vi "BinSearchVIwarmcold.vi"(8 "X0":sgl=0.5, 11 "Ring":i16(ring) items=["Warm", "Cold"]) -> (3 "Xpot":sgl)   [LabVIEW 2019]
uses:
  <vilib>/Platform/TimedLoop/XDataNode/timing_clust.ctl
  <vilib>/Platform/TimedLoop/XDataNode/nitl_modes.ctl
  <vilib>/Platform/TimedLoop/XDataNode/wakeup.ctl
  <vilib>/rvi/Emulation/niFpgaGetClockAttributes.vi
  <vilib>/rvi/Emulation/niFpgaSctlEmulationGetInTimedLoop.vi
  <vilib>/rvi/Emulation/niFpgaEmulationReportErrorSimple.vi
  <vilib>/rvi/Emulation/niFpgaCriticalErrorInLSC.vi
  <vilib>/Platform/TimedLoop/XDataNode/XDataNode.xnode
  <vilib>/Platform/TimedLoop/XDataNode/XDNodeRunTimeDep.lvlib
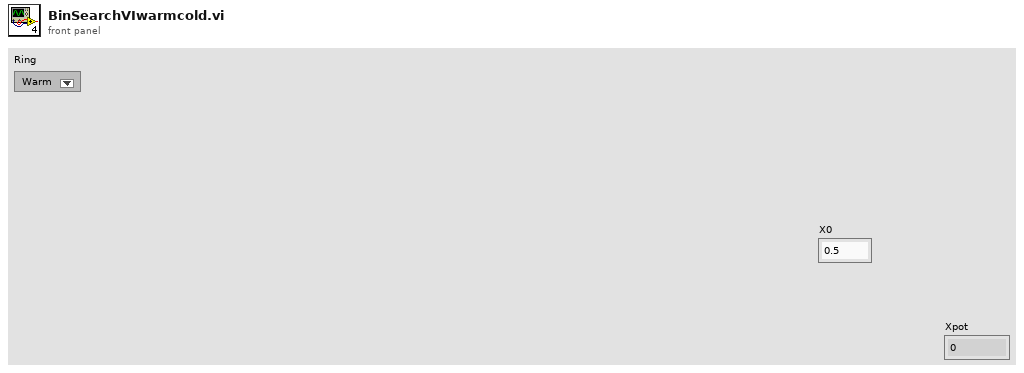
[diagram p1: front panel]
types:
  T1 = typedef "XDNodeRunTimeDep.lvlib/timing_clust.ctl" = cluster{"Expected End [f-1]":u64, "Actual End [f-1]":u64, "Finished Late? [f-1]":bool, "Expected End [i-1]":u64, "Actual End [i-1]":u64, "Finished Late? [i-1]":bool, "Expected Start [i]":u64, "Actual Start [i]":u64, "Expected Start [f]":u64, "Actual Start [f]":u64, "Source Name":string, "Structure Name":string, "Period":i64, "Deadline":i64, "Offset":i64, "Start":i64, "Priority":i32, "Timeout":i32, "Mode":T2, "Wakeup Reason":T3, "Error":errorcluster, "Source Type":string, "Secondary Source Type":string, "Global End Time":u64, "Global Start Time":u64, "Frame Duration":u64, "Iteration Duration":u64, "Assigned CPU":i32, "I/O Scan Engine Mode":u32}
  T2 = typedef "XDNodeRunTimeDep.lvlib/nitl_modes.ctl" = enum32{"No Change", "Process missed periods, maintain original phase", "Discard missed periods, maintain original phase", "Process missed periods, ignore original phase", "Discard missed periods, ignore original phase"}
  T3 = typedef "XDNodeRunTimeDep.lvlib/wakeup.ctl" = enum32{"Normal", "Aborted", "Asynchronous wakeup", "Timing source error", "Timed loop error", "Timeout"}
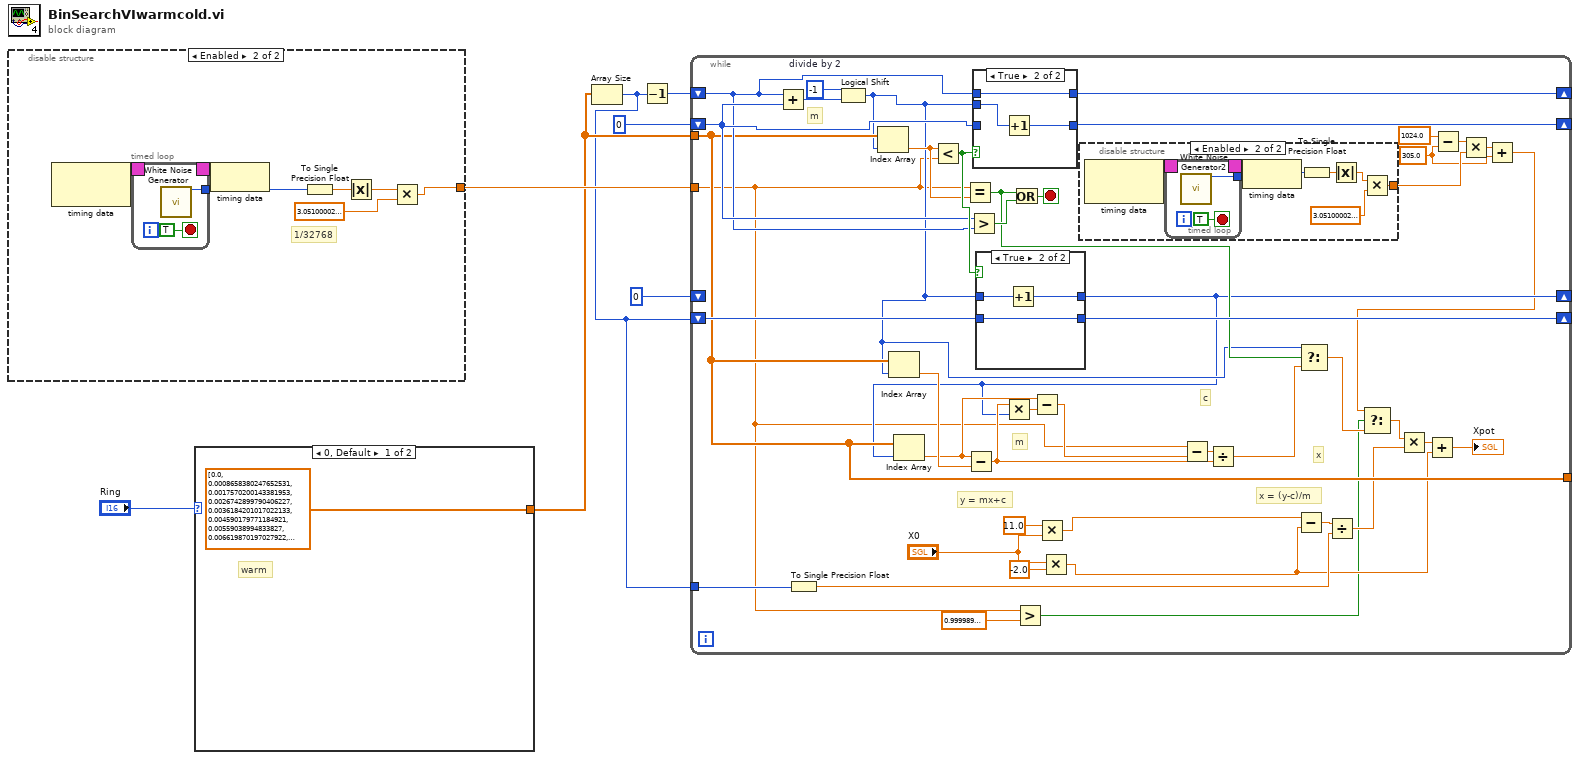
[diagram p0: block diagram]
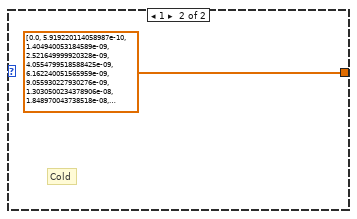
[diagram p2: hidden frame]
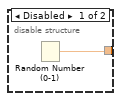
[diagram p3: hidden frame]
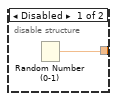
[diagram p4: hidden frame]
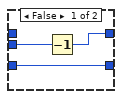
[diagram p6: hidden frame]
diagram:
  n1 = disable-structure shown="Enabled" {
    disable-tunnel: [w8 w11] -> w4
    frame Disabled {
      n2 = Random Number (0-1)() -> (number: 0 to 1=w8:dbl)
    }
    frame Enabled {
      # "1/32768"
      n3 = node-c288() -> (w10:T1)  [unwired: 1 in]
      n4 = timed-loop {
        timing: w10 -> [_]
        timing-out: [_] -> w9
        tunnel: [w17] -> w15
        stop <- TRUE stop-if-true
        n5 = call "White Noise Generator"() -> ("white noise out"=w17:i16)  [unwired: 15 in]
      }
      n6 = node-c288(w9) -> ()
      n7 = To Single Precision Float(number=w15) -> (single precision float=w13:sgl)
      n8 = Absolute Value(x=w13) -> (abs(x)=w12:sgl)
      n9 = Multiply(x=w12, y=sgl 3.051e-05) -> (x*y=w11:sgl)
    }
  }
  n10 = case shown="0, Default" "Ring" {
    tunnel: [sgl[] [0.0, 0.000865838, 0.00175702, 0.00267429, 0.00361842, 0.00459018, 0.00559039, 0.00661987, 0.0076795, 0.00877014, 0.00989271, 0.0110481, 0.0122374, 0.0134615, 0.0147214, 0.0160181, 0.0173529, 0.0187267, 0.0201407, 0.0215961, 0.0230942, 0.0246361, 0.0262231, 0.0278565, 0.0295378, 0.0312683, 0.0330498, 0.0348832, 0.0367683, 0.0387052, 0.0406935, 0.0427329, 0.044823, 0.0469636, 0.0491541, 0.0513939, 0.0536825, 0.0560193, 0.0584036, 0.0608346, 0.0633115, 0.0658336, 0.0683999, 0.0710095, 0.0736616, 0.076355, 0.0790889, 0.0818621, 0.0846736, 0.0875224, 0.0904072, 0.0933269, 0.0962805, 0.0992667, 0.102284, 0.105332, 0.108409, 0.111514, 0.114646, 0.117803, 0.120985, 0.12419, 0.127416, 0.130664, 0.133931, 0.137217, 0.14052, 0.143839, 0.147174, 0.150523, 0.153884, 0.157258, 0.160643, 0.164038, 0.167441, 0.170853, 0.174272, 0.177698, 0.181129, 0.184564, 0.188003, 0.191445, 0.19489, 0.198336, 0.201783, 0.20523, 0.208676, 0.212122, 0.215565, 0.219007, 0.222446, 0.225881, 0.229313, 0.232741, 0.236164, 0.239582, 0.242995, 0.246402, 0.249804, 0.253199, 0.256587, 0.259969, 0.263344, 0.266712, 0.270072, 0.273425, 0.276771, 0.280108, 0.283438, 0.286761, 0.290075, 0.293381, 0.29668, 0.29997, 0.303253, 0.306527, 0.309795, 0.313054, 0.316306, 0.31955, 0.322787, 0.326016, 0.329239, 0.332454, 0.335663, 0.338865, 0.34206, 0.34525, 0.348433, 0.351611, 0.354783, 0.35795, 0.361111, 0.364268, 0.36742, 0.370568, 0.373713, 0.376853, 0.37999, 0.383123, 0.386254, 0.389383, 0.392509, 0.395634, 0.398756, 0.401878, 0.404999, 0.408119, 0.411239, 0.414359, 0.41748, 0.420602, 0.423725, 0.426849, 0.429976, 0.433104, 0.436236, 0.43937, 0.442508, 0.44565, 0.448796, 0.451946, 0.455101, 0.458262, 0.461428, 0.4646, 0.467779, 0.470964, 0.474157, 0.477357, 0.480565, 0.483782, 0.487007, 0.490241, 0.493484, 0.496738, 0.500001, 0.503275, 0.506559, 0.509855, 0.513162, 0.516481, 0.519812, 0.523156, 0.526513, 0.529882, 0.533265, 0.536662, 0.540073, 0.543498, 0.546938, 0.550393, 0.553862, 0.557348, 0.560848, 0.564365, 0.567898, 0.571446, 0.575012, 0.578594, 0.582192, 0.585808, 0.58944, 0.59309, 0.596757, 0.600441, 0.604143, 0.607862, 0.611598, 0.615352, 0.619123, 0.622911, 0.626717, 0.630539, 0.634379, 0.638235, 0.642109, 0.645998, 0.649904, 0.653825, 0.657762, 0.661715, 0.665682, 0.669664, 0.67366, 0.67767, 0.681692, 0.685727, 0.689775, 0.693833, 0.697902, 0.701981, 0.70607, 0.710167, 0.714272, 0.718383, 0.722501, 0.726624, 0.73075, 0.73488, 0.739012, 0.743145, 0.747277, 0.751408, 0.755537, 0.759661, 0.763781, 0.767894, 0.772, 0.776096, 0.780182, 0.784256, 0.788316, 0.792362, 0.79639, 0.800401, 0.804392, 0.808362, 0.812309, 0.816232, 0.820128, 0.823996, 0.827836, 0.831643, 0.835419, 0.839159, 0.842864, 0.846531, 0.850159, 0.853745, 0.857289, 0.860789, 0.864243, 0.86765, 0.871009, 0.874317, 0.877573, 0.880777, 0.883927, 0.887021, 0.890059, 0.893039, 0.89596, 0.898821, 0.901622, 0.904361, 0.907038, 0.909651, 0.912201, 0.914687, 0.917108, 0.919465, 0.921755, 0.92398, 0.926142, 0.928243, 0.930284, 0.932267, 0.934193, 0.936065, 0.937883, 0.93965, 0.941366, 0.943034, 0.944654, 0.946228, 0.947757, 0.949243, 0.950687, 0.952089, 0.953452, 0.954776, 0.956062, 0.957312, 0.958526, 0.959705, 0.960851, 0.961965, 0.963047, 0.964098, 0.965119, 0.966111, 0.967075, 0.968011, 0.968921, 0.969805, 0.970664, 0.971498, 0.972309, 0.973096, 0.973861, 0.974605, 0.975327, 0.976029, 0.976711, 0.977373, 0.978016, 0.978642, 0.979249, 0.979839, 0.980413, 0.98097, 0.981511, 0.982037, 0.982548, 0.983044, 0.983527, 0.983995, 0.98445, 0.984893, 0.985322, 0.98574, 0.986145, 0.986539, 0.986922, 0.987294, 0.987656, 0.988007, 0.988348, 0.988679, 0.989001, 0.989314, 0.989618, 0.989913, 0.9902, 0.990479, 0.99075, 0.991013, 0.991268, 0.991517, 0.991758, 0.991992, 0.99222, 0.992441, 0.992656, 0.992865, 0.993068, 0.993265, 0.993457, 0.993643, 0.993824, 0.993999, 0.99417, 0.994336, 0.994497, 0.994654, 0.994806, 0.994953, 0.995097, 0.995236, 0.995372, 0.995504, 0.995631, 0.995756, 0.995876, 0.995994, 0.996108, 0.996218, 0.996326, 0.996431, 0.996532, 0.996631, 0.996727, 0.99682, 0.99691, 0.996998, 0.997083, 0.997166, 0.997247, 0.997325, 0.997401, 0.997475, 0.997547, 0.997617, 0.997685, 0.997751, 0.997815, 0.997877, 0.997937, 0.997996, 0.998053, 0.998108, 0.998162, 0.998214, 0.998265, 0.998314, 0.998362, 0.998409, 0.998454, 0.998498, 0.998541, 0.998583, 0.998623, 0.998662, 0.9987, 0.998737, 0.998773, 0.998808, 0.998842, 0.998875, 0.998907, 0.998938, 0.998968, 0.998998, 0.999026, 0.999054, 0.999081, 0.999107, 0.999132, 0.999157, 0.999181, 0.999204, 0.999227, 0.999249, 0.99927, 0.999291, 0.999311, 0.999331, 0.99935, 0.999369, 0.999387, 0.999404, 0.999421, 0.999438, 0.999454, 0.999469, 0.999484, 0.999499, 0.999513, 0.999527, 0.999541, 0.999554, 0.999566, 0.999579, 0.999591, 0.999602, 0.999614, 0.999625, 0.999635, 0.999646, 0.999656, 0.999666, 0.999675, 0.999684, 0.999693, 0.999702, 0.999711, 0.999719, 0.999727, 0.999735, 0.999742, 0.99975, 0.999757, 0.999764, 0.99977, 0.999777, 0.999783, 0.999789, 0.999795, 0.999801, 0.999807, 0.999812, 0.999818, 0.999823, 0.999828, 0.999833, 0.999838, 0.999842, 0.999847, 0.999851, 0.999856, 0.99986, 0.999864, 0.999867, 0.999871, 0.999875, 0.999879, 0.999882, 0.999885, 0.999889, 0.999892, 0.999895, 0.999898, 0.999901, 0.999904, 0.999906, 0.999909, 0.999912, 0.999914, 0.999917, 0.999919, 0.999921, 0.999924, 0.999926, 0.999928, 0.99993, 0.999932, 0.999934, 0.999936, 0.999938, 0.99994, 0.999941, 0.999943, 0.999945, 0.999946, 0.999948, 0.999949, 0.999951, 0.999952, 0.999954, 0.999955, 0.999956, 0.999958, 0.999959, 0.99996, 0.999961, 0.999962, 0.999963, 0.999964, 0.999965, 0.999966, 0.999967, 0.999968, 0.999969, 0.99997, 0.999971, 0.999972, 0.999973, 0.999973, 0.999974, 0.999975, 0.999976, 0.999976, 0.999977, 0.999978, 0.999978, 0.999979, 0.99998, 0.99998, 0.999981, 0.999981, 0.999982, 0.999983, 0.999983, 0.999984, 0.999984, 0.999985, 0.999985, 0.999985, 0.999986, 0.999986, 0.999987, 0.999987, 0.999988, 0.999988, 0.999988, 0.999989, 0.999989, 0.999989, 0.99999, 0.99999, 0.99999, 0.999991, 0.999991, 0.999991, 0.999991, 0.999992, 0.999992, 0.999992, 0.999992, 0.999993, 0.999993, 0.999993, 0.999993, 0.999994, 0.999994, 0.999994, 0.999994, 0.999994, 0.999994, 0.999995, 0.999995, 0.999995, 0.999995, 0.999995, 0.999996, 0.999996, 0.999996, 0.999996, 0.999996, 0.999996, 0.999996, 0.999996, 0.999997, 0.999997, 0.999997, 0.999997, 0.999997, 0.999997, 0.999997, 0.999997, 0.999997, 0.999998, 0.999998, 0.999998, 0.999998, 0.999998, 0.999998, 0.999998, 0.999998, 0.999998, 0.999998, 0.999998, 0.999998, 0.999998, 0.999998, 0.999999, 0.999999, 0.999999, 0.999999, 0.999999, 0.999999, 0.999999, 0.999999, 0.999999, 0.999999, 0.999999, 0.999999, 0.999999, 0.999999, 0.999999, 0.999999, 0.999999, 1.0, 1.0, 1.0, 1.0, 1.0, 1.0, 1.0, 1.0, 1.0, 1.0, 1.0, 1.0, 1.0, 1.0, 1.0, 1.0, 1.0, 1.0, 1.0, 1.0, 1.0, 1.0, 1.0, 1.0, 1.0, 1.0, 1.0, 1.0, 1.0, 1.0, 1.0, 1.0, 1.0, 1.0, 1.0, 1.0, 1.0, 1.0, 1.0, 1.0, 1.0, 1.0, 1.0, 1.0, 1.0, 1.0, 1.0, 1.0, 1.0, 1.0, 1.0, 1.0, 1.0, 1.0, 1.0, 1.0, 1.0, 1.0, 1.0, 1.0, 1.0, 1.0, 1.0, 1.0, 1.0, 1.0, 1.0, 1.0, 1.0, 1.0, 1.0, 1.0, 1.0, 1.0, 1.0, 1.0, 1.0, 1.0, 1.0, 1.0, 1.0, 1.0, 1.0, 1.0, 1.0, 1.0, 1.0, 1.0, 1.0, 1.0, 1.0, 1.0, 1.0, 1.0, 1.0, 1.0, 1.0, 1.0, 1.0, 1.0, 1.0, 1.0, 1.0, 1.0, 1.0, 1.0, 1.0, 1.0, 1.0, 1.0, 1.0, 1.0, 1.0, 1.0, 1.0, 1.0, 1.0, 1.0, 1.0, 1.0, 1.0, 1.0, 1.0, 1.0, 1.0, 1.0, 1.0, 1.0, 1.0, 1.0, 1.0, 1.0, 1.0, 1.0, 1.0, 1.0, 1.0, 1.0, 1.0, 1.0, 1.0, 1.0, 1.0, 1.0, 1.0, 1.0, 1.0, 1.0, 1.0, 1.0, 1.0, 1.0, 1.0, 1.0, 1.0, 1.0, 1.0, 1.0, 1.0, 1.0, 1.0, 1.0, 1.0, 1.0, 1.0, 1.0, 1.0, 1.0, 1.0, 1.0, 1.0, 1.0, 1.0, 1.0, 1.0, 1.0, 1.0, 1.0, 1.0, 1.0, 1.0, 1.0, 1.0, 1.0, 1.0, 1.0, 1.0, 1.0, 1.0, 1.0, 1.0, 1.0, 1.0, 1.0, 1.0, 1.0, 1.0, 1.0, 1.0, 1.0, 1.0, 1.0, 1.0, 1.0, 1.0, 1.0, 1.0, 1.0, 1.0, 1.0, 1.0, 1.0, 1.0, 1.0, 1.0, 1.0, 1.0, 1.0, 1.0, 1.0, 1.0, 1.0, 1.0, 1.0, 1.0, 1.0, 1.0, 1.0, 1.0, 1.0, 1.0, 1.0, 1.0, 1.0, 1.0, 1.0, 1.0, 1.0, 1.0, 1.0, 1.0, 1.0, 1.0, 1.0, 1.0, 1.0, 1.0, 1.0, 1.0, 1.0, 1.0, 1.0, 1.0, 1.0, 1.0, 1.0, 1.0, 1.0, 1.0, 1.0, 1.0, 1.0, 1.0, 1.0, 1.0, 1.0, 1.0, 1.0, 1.0, 1.0, 1.0, 1.0, 1.0, 1.0, 1.0, 1.0, 1.0, 1.0, 1.0, 1.0, 1.0, 1.0, 1.0, 1.0, 1.0, 1.0, 1.0, 1.0, 1.0, 1.0, 1.0, 1.0, 1.0, 1.0, 1.0, 1.0, 1.0, 1.0, 1.0, 1.0, 1.0, 1.0, 1.0, 1.0, 1.0, 1.0, 1.0, 1.0, 1.0, 1.0, 1.0, 1.0, 1.0, 1.0, 1.0, 1.0, 1.0, 1.0, 1.0, 1.0, 1.0, 1.0, 1.0, 1.0, 1.0, 1.0, 1.0, 1.0, 1.0, 1.0, 1.0, 1.0, 1.0, 1.0, 1.0, 1.0, 1.0, 1.0, 1.0, 1.0, 1.0, 1.0, 1.0, 1.0, 1.0, 1.0, 1.0, 1.0, 1.0, 1.0, 1.0] ("Init Data Out") sgl[] [0.0, 5.91922e-10, 1.40494e-09, 2.52165e-09, 4.05548e-09, 6.16224e-09, 9.05593e-09, 1.30305e-08, 1.84897e-08, 2.5988e-08, 3.62872e-08, 5.04334e-08, 6.98637e-08, 9.65517e-08, 1.33208e-07, 1.83557e-07, 2.52713e-07, 3.47701e-07, 4.78169e-07, 6.5737e-07, 9.03508e-07, 1.24159e-06, 1.70595e-06, 2.34376e-06, 3.21981e-06, 4.42309e-06, 6.07913e-06, 8.34909e-06, 1.14315e-05, 1.55788e-05, 2.11084e-05, 2.84159e-05, 3.79887e-05, 5.04218e-05, 6.64346e-05, 8.68874e-05, 0.0001128, 0.00014537, 0.000185987, 0.000236255, 0.000297998, 0.000373279, 0.000464407, 0.000573936, 0.000704673, 0.000859665, 0.00104219, 0.00125576, 0.00150404, 0.00179088, 0.00212026, 0.00249623, 0.00292289, 0.00340431, 0.00394449, 0.00454732, 0.0052165, 0.00595547, 0.0067674, 0.00765509, 0.00862095, 0.00966693, 0.0107945, 0.0120047, 0.0132978, 0.0146739, 0.0161321, 0.0176713, 0.0192896, 0.0209848, 0.022754, 0.024594, 0.026501, 0.028471, 0.0304993, 0.0325814, 0.0347122, 0.0368865, 0.039099, 0.0413443, 0.043617, 0.0459116, 0.0482228, 0.0505453, 0.052874, 0.0552039, 0.0575303, 0.0598487, 0.0621549, 0.0644448, 0.0667148, 0.0689614, 0.0711815, 0.0733723, 0.0755313, 0.0776562, 0.0797451, 0.0817963, 0.0838084, 0.0857803, 0.0877111, 0.0896, 0.0914467, 0.0932509, 0.0950124, 0.0967315, 0.0984082, 0.100043, 0.101637, 0.103189, 0.104702, 0.106176, 0.107611, 0.109009, 0.11037, 0.111696, 0.112988, 0.114247, 0.115474, 0.11667, 0.117836, 0.118974, 0.120085, 0.121169, 0.122229, 0.123265, 0.124278, 0.12527, 0.126241, 0.127193, 0.128127, 0.129043, 0.129944, 0.13083, 0.131702, 0.132561, 0.133408, 0.134244, 0.13507, 0.135887, 0.136696, 0.137498, 0.138293, 0.139084, 0.13987, 0.140653, 0.141434, 0.142213, 0.142992, 0.143771, 0.144551, 0.145334, 0.146121, 0.146911, 0.147708, 0.14851, 0.149321, 0.15014, 0.150968, 0.151808, 0.152661, 0.153527, 0.154408, 0.155305, 0.15622, 0.157155, 0.158111, 0.159089, 0.160092, 0.161121, 0.162178, 0.163266, 0.164387, 0.165542, 0.166735, 0.167968, 0.169244, 0.170566, 0.171936, 0.173358, 0.174836, 0.176373, 0.177974, 0.179641, 0.181381, 0.183196, 0.185093, 0.187077, 0.189152, 0.191326, 0.193604, 0.195992, 0.198498, 0.201128, 0.203892, 0.206796, 0.209848, 0.213059, 0.216438, 0.219993, 0.223736, 0.227676, 0.231826, 0.236196, 0.240798, 0.245644, 0.250748, 0.256121, 0.261778, 0.26773, 0.273992, 0.280577, 0.287499, 0.294771, 0.302406, 0.310417, 0.318816, 0.327616, 0.336826, 0.346458, 0.356519, 0.367018, 0.377961, 0.389351, 0.401192, 0.413483, 0.426223, 0.439407, 0.453028, 0.467075, 0.481535, 0.496392, 0.511624, 0.527209, 0.543119, 0.559324, 0.57579, 0.592479, 0.60935, 0.62636, 0.643461, 0.660604, 0.677739, 0.694811, 0.711768, 0.728553, 0.745111, 0.761389, 0.777333, 0.792891, 0.808013, 0.822655, 0.836773, 0.850328, 0.863287, 0.875622, 0.887308, 0.898329, 0.908671, 0.91833, 0.927305, 0.935601, 0.943229, 0.950204, 0.956548, 0.962284, 0.96744, 0.972049, 0.976142, 0.979754, 0.982923, 0.985684, 0.988074, 0.990129, 0.991883, 0.993371, 0.994623, 0.995668, 0.996536, 0.99725, 0.997832, 0.998305, 0.998684, 0.998986, 0.999225, 0.999412, 0.999558, 0.99967, 0.999755, 0.999819, 0.999868, 0.999904, 0.99993, 0.999949, 0.999963, 0.999973, 0.99998, 0.999986, 0.99999, 0.999993, 0.999995, 0.999996, 0.999997, 0.999998, 0.999999, 0.999999, 0.999999, 1.0, 1.0, 1.0, 1.0, 1.0, 1.0, 1.0, 1.0, 1.0, 1.0, 1.0, 1.0, 1.0, 1.0, 1.0, 1.0, 1.0, 1.0, 1.0, 1.0, 1.0, 1.0, 1.0, 1.0, 1.0, 1.0, 1.0, 1.0, 1.0, 1.0, 1.0, 1.0, 1.0, 1.0, 1.0, 1.0, 1.0, 1.0, 1.0, 1.0, 1.0, 1.0, 1.0, 1.0, 1.0, 1.0, 1.0, 1.0, 1.0, 1.0, 1.0, 1.0, 1.0, 1.0, 1.0, 1.0, 1.0, 1.0, 1.0, 1.0, 1.0, 1.0, 1.0, 1.0, 1.0, 1.0, 1.0, 1.0, 1.0, 1.0, 1.0, 1.0, 1.0, 1.0, 1.0, 1.0, 1.0, 1.0, 1.0, 1.0, 1.0, 1.0, 1.0, 1.0, 1.0, 1.0, 1.0, 1.0, 1.0, 1.0, 1.0, 1.0, 1.0, 1.0, 1.0, 1.0, 1.0, 1.0, 1.0, 1.0, 1.0, 1.0, 1.0, 1.0, 1.0, 1.0, 1.0, 1.0, 1.0, 1.0, 1.0, 1.0, 1.0, 1.0, 1.0, 1.0, 1.0, 1.0, 1.0, 1.0, 1.0, 1.0, 1.0, 1.0, 1.0, 1.0, 1.0, 1.0, 1.0, 1.0, 1.0, 1.0, 1.0, 1.0, 1.0, 1.0, 1.0, 1.0, 1.0, 1.0, 1.0, 1.0, 1.0, 1.0, 1.0, 1.0, 1.0, 1.0, 1.0, 1.0, 1.0, 1.0, 1.0, 1.0, 1.0, 1.0, 1.0, 1.0, 1.0, 1.0, 1.0, 1.0, 1.0, 1.0, 1.0, 1.0, 1.0, 1.0, 1.0, 1.0, 1.0, 1.0, 1.0, 1.0, 1.0, 1.0, 1.0, 1.0, 1.0, 1.0, 1.0, 1.0, 1.0, 1.0, 1.0, 1.0, 1.0, 1.0, 1.0, 1.0, 1.0, 1.0, 1.0, 1.0, 1.0, 1.0, 1.0, 1.0, 1.0, 1.0, 1.0, 1.0, 1.0, 1.0, 1.0, 1.0, 1.0, 1.0, 1.0, 1.0, 1.0, 1.0, 1.0, 1.0, 1.0, 1.0, 1.0, 1.0, 1.0, 1.0, 1.0, 1.0, 1.0, 1.0, 1.0, 1.0, 1.0, 1.0, 1.0, 1.0, 1.0, 1.0, 1.0, 1.0, 1.0, 1.0, 1.0, 1.0, 1.0, 1.0, 1.0, 1.0, 1.0, 1.0, 1.0, 1.0, 1.0, 1.0, 1.0, 1.0, 1.0, 1.0, 1.0, 1.0, 1.0, 1.0, 1.0, 1.0, 1.0, 1.0, 1.0, 1.0, 1.0, 1.0, 1.0, 1.0, 1.0, 1.0, 1.0, 1.0, 1.0, 1.0, 1.0, 1.0, 1.0, 1.0, 1.0, 1.0, 1.0, 1.0, 1.0, 1.0, 1.0, 1.0, 1.0, 1.0, 1.0, 1.0, 1.0, 1.0, 1.0, 1.0, 1.0, 1.0, 1.0, 1.0, 1.0, 1.0, 1.0, 1.0, 1.0, 1.0, 1.0, 1.0, 1.0, 1.0, 1.0, 1.0, 1.0, 1.0, 1.0, 1.0, 1.0, 1.0, 1.0, 1.0, 1.0, 1.0, 1.0, 1.0, 1.0, 1.0, 1.0, 1.0, 1.0, 1.0, 1.0, 1.0, 1.0, 1.0, 1.0, 1.0, 1.0, 1.0, 1.0, 1.0, 1.0, 1.0, 1.0, 1.0, 1.0, 1.0, 1.0, 1.0, 1.0, 1.0, 1.0, 1.0, 1.0, 1.0, 1.0, 1.0, 1.0, 1.0, 1.0, 1.0, 1.0, 1.0, 1.0, 1.0, 1.0, 1.0, 1.0, 1.0, 1.0, 1.0, 1.0, 1.0, 1.0, 1.0, 1.0, 1.0, 1.0, 1.0, 1.0, 1.0, 1.0, 1.0, 1.0, 1.0, 1.0, 1.0, 1.0, 1.0, 1.0, 1.0, 1.0, 1.0, 1.0, 1.0, 1.0, 1.0, 1.0, 1.0, 1.0, 1.0, 1.0, 1.0, 1.0, 1.0, 1.0, 1.0, 1.0, 1.0, 1.0, 1.0, 1.0, 1.0, 1.0, 1.0, 1.0, 1.0, 1.0, 1.0, 1.0, 1.0, 1.0, 1.0, 1.0, 1.0, 1.0, 1.0, 1.0, 1.0, 1.0, 1.0, 1.0, 1.0, 1.0, 1.0, 1.0, 1.0, 1.0, 1.0, 1.0, 1.0, 1.0, 1.0, 1.0, 1.0, 1.0, 1.0, 1.0, 1.0, 1.0, 1.0, 1.0, 1.0, 1.0, 1.0, 1.0, 1.0, 1.0, 1.0, 1.0, 1.0, 1.0, 1.0, 1.0, 1.0, 1.0, 1.0, 1.0, 1.0, 1.0, 1.0, 1.0, 1.0, 1.0, 1.0, 1.0, 1.0, 1.0, 1.0, 1.0, 1.0, 1.0, 1.0, 1.0, 1.0, 1.0, 1.0, 1.0, 1.0, 1.0, 1.0, 1.0, 1.0, 1.0, 1.0, 1.0, 1.0, 1.0, 1.0, 1.0, 1.0, 1.0, 1.0, 1.0, 1.0, 1.0, 1.0, 1.0, 1.0, 1.0, 1.0, 1.0, 1.0, 1.0, 1.0, 1.0, 1.0, 1.0, 1.0, 1.0, 1.0, 1.0, 1.0, 1.0, 1.0, 1.0, 1.0, 1.0, 1.0, 1.0, 1.0, 1.0, 1.0, 1.0, 1.0, 1.0, 1.0, 1.0, 1.0, 1.0, 1.0, 1.0, 1.0, 1.0, 1.0, 1.0, 1.0, 1.0, 1.0, 1.0, 1.0, 1.0, 1.0, 1.0, 1.0, 1.0, 1.0, 1.0, 1.0, 1.0, 1.0, 1.0, 1.0, 1.0, 1.0, 1.0, 1.0, 1.0, 1.0, 1.0, 1.0, 1.0, 1.0, 1.0, 1.0, 1.0, 1.0, 1.0, 1.0, 1.0, 1.0, 1.0, 1.0, 1.0, 1.0, 1.0, 1.0, 1.0, 1.0, 1.0, 1.0, 1.0, 1.0, 1.0, 1.0, 1.0, 1.0, 1.0, 1.0, 1.0, 1.0, 1.0, 1.0, 1.0, 1.0, 1.0, 1.0, 1.0, 1.0, 1.0, 1.0, 1.0, 1.0, 1.0, 1.0, 1.0, 1.0, 1.0, 1.0, 1.0, 1.0, 1.0, 1.0, 1.0, 1.0, 1.0, 1.0, 1.0, 1.0, 1.0, 1.0, 1.0, 1.0, 1.0, 1.0, 1.0, 1.0, 1.0, 1.0, 1.0, 1.0, 1.0, 1.0, 1.0, 1.0, 1.0, 1.0, 1.0, 1.0, 1.0, 1.0, 1.0, 1.0, 1.0, 1.0, 1.0, 1.0, 1.0, 1.0, 1.0, 1.0, 1.0, 1.0, 1.0, 1.0, 1.0, 1.0, 1.0, 1.0, 1.0, 1.0, 1.0, 1.0, 1.0, 1.0, 1.0, 1.0, 1.0, 1.0, 1.0, 1.0, 1.0, 1.0, 1.0, 1.0, 1.0, 1.0, 1.0, 1.0, 1.0, 1.0, 1.0, 1.0, 1.0, 1.0, 1.0, 1.0, 1.0, 1.0, 1.0, 1.0, 1.0, 1.0, 1.0, 1.0, 1.0, 1.0, 1.0, 1.0, 1.0, 1.0, 1.0, 1.0, 1.0, 1.0, 1.0, 1.0, 1.0, 1.0, 1.0, 1.0, 1.0] ("Init Data Out")] -> w2
    frame 0, Default {
      # "warm"
    }
    frame 1 {
      # "Cold"
    }
  }
  n11 = Array Size(array=w2) -> (size(s)=w1:i32)
  n12 = Decrement(x=w1) -> (x-1=w5:i32)
  n13 = while {
    tunnel: w2 -> [w55]
    tunnel: w4 -> [w34]
    shift-right: [w67] -> _
    shift-left: w5 -> [w58]
    shift-right: [w63] -> _
    shift-left: 0 -> [w59]
    shift-right: [w46] -> _
    shift-left: 0 -> [_]
    shift-right: [w60] -> _
    shift-left: w1 -> [w61]
    tunnel: [w55] -> _
    tunnel: w1 -> [w40]
    stop <- w65 stop-if-true
    w27 = sgl 305.0 ("y")
    w68 = -1  # divide by 2
    # "x"
    # "x = (y-c)/m"
    # "c"
    # "m"
    # "y = mx+c"
    # "m"
    n14 = Add(x=w58, y=w59) -> (x+y=w64:i32)
    n15 = To Single Precision Float(number=w40) -> (single precision float=w39:sgl)
    n16 = Logical Shift(y=w68, x=w64) -> (x << y=w53:i32)
    n17 = Index Array(array=w55, index=w53) -> (element=w57:sgl)
    n18 = Index Array(array=w55, index=w53) -> (element=w56:sgl)
    n19 = Less?(x=w57, y=w34) -> (x < y?=w62:bool)
    n20 = Equal?(x=w34, y=w57) -> (x = y?=w54:bool)
    n21 = Greater?(x=w59, y=w58) -> (0:w66:bool)
    n22 = case shown="True" w62 {
      tunnel: w53 -> [w90 w93]
      tunnel: [w89 w91] -> w67
      tunnel: w59 -> [w88 _]
      tunnel: [w88 w92] -> w63
      tunnel: w58 -> [_ w91]
      frame False {
        n23 = Decrement(x=w90) -> (x-1=w89:i32)
      }
      frame True {
        n24 = Increment(x=w93) -> (x+1=w92:i32)
      }
    }
    n25 = case shown="True" w62 {
      tunnel: w53 -> [w84 w87]
      tunnel: [w83 w86] -> w46
      tunnel: w61 -> [w83 w85]
      tunnel: [w84 w85] -> w60
      frame False {
      }
      frame True {
        n26 = Increment(x=w87) -> (x+1=w86:i32)
      }
    }
    n27 = Index Array(array=w55, index=w46) -> (element=w51:sgl)
    n28 = Subtract(x=w51, y=w56) -> (x-y=w48:sgl)
    n29 = Multiply(x=w48, y=w46) -> (x*y=w52:sgl)
    n30 = Or(x=w54, y=w66) -> (x .or. y?=w65:bool)
    n31 = Greater?(x=w34, y=sgl 0.99999) -> (0:w24:bool)
    n32 = Subtract(x=w51, y=w52) -> (x-y=w50:sgl)
    n33 = Multiply(x=sgl 11.0, y="X0") -> (x*y=w43:sgl)
    n34 = Multiply(x="X0", y=sgl -2.0) -> (x*y=w37:sgl)
    n35 = disable-structure shown="Enabled" {
      disable-tunnel: [w69 w72] -> w29
      frame Disabled {
        n36 = Random Number (0-1)() -> (number: 0 to 1=w69:dbl)
      }
      frame Enabled {
        n37 = node-c288() -> (w71:T1)  [unwired: 1 in]
        n38 = timed-loop {
          timing: w71 -> [_]
          timing-out: [_] -> w70
          tunnel: [w78] -> w76
          stop <- TRUE stop-if-true
          n39 = call "White Noise Generator2"() -> ("white noise out"=w78:i16)  [unwired: 15 in]
        }
        n40 = node-c288(w70) -> ()
        n41 = To Single Precision Float(number=w76) -> (single precision float=w74:sgl)
        n42 = Absolute Value(x=w74) -> (abs(x)=w73:sgl)
        n43 = Multiply(x=w73, y=sgl 3.051e-05) -> (x*y=w72:sgl)
      }
    }
    n44 = Subtract(x=w34, y=w50) -> (x-y=w49:sgl)
    n45 = Divide(x=w49, y=w48) -> (x/y=w47:sgl)
    n46 = Subtract(x=w43, y=w37) -> (x-y=w42:sgl)
    n47 = Select(t=w53, s=w54, f=w47) -> (s? t:f=w32:sgl)
    n48 = Divide(x=w42, y=w39) -> (x/y=w41:sgl)
    n49 = Subtract(x=sgl 1024.0, y=w27) -> (x-y=w30:sgl)
    n50 = Multiply(x=w30, y=w29) -> (x*y=w28:sgl)
    n51 = Add(x=w28, y=w27) -> (x+y=w25:sgl)
    n52 = Select(t=w25, s=w24, f=w32) -> (s? t:f=w26:sgl)
    n53 = Multiply(x=w26, y=w41) -> (x*y=w38:sgl)
    n54 = Add(x=w38, y=w37) -> (x+y=→"Xpot":sgl)
  }
